vi "ADIS16448 IMU Example.vi"() -> ()   [LabVIEW 2019]
uses:
  <vilib>/Utility/RT CPU Load.ctl
  ADIS16448Lib/Typedef/ADIS16448 Hardware Configuration.ctl
  <vilib>/Rock Robotics/WPI/SPI/WPI_SPIMode.ctl
  <vilib>/Rock Robotics/SystemInterfaces/DIO/FPGA_DIOChannel.ctl
  <vilib>/Rock Robotics/SystemInterfaces/spilib/spi_bus.ctl
  <vilib>/NI_Real-Time Target Support.lvlib
panel:
  out "Accelerometers":T1(graph)
  out "IMU Detected?":bool
  in  "Calibration Time (sec)":u32=4
  in  "Hardware Config":T2={"SPI Clock Rate (Hz)"=1000000.0, "IMU SPI Mode (3)"=enum."Mode 3 (Clk Idle High,Sample on Trailing)", "IMU Reset Pin"=enum."DIO MXP 8", "IMU SPI Bus"=enum."SPI MXP", "IMU Data Ready Pin"=enum."DIO MXP 0", "Stall Config"={"Pow2BytesPerRead"=255, "StallTicks"=1000, "CsToSclkTicks"=5}, "IMU Status LED Pin"=enum."DIO MXP 9"}
  in  "Recalibrate?":bool
  in  "Reset?":bool
  out "Integrated Gyro Angle":T1(graph)
  out "Calibrated?":bool
  in  "Set Cal Time":bool
  out "CPU loads":T6[](array[typedef]) {"ISR (%)" format="%#.2f"; "Idle (%)" format="%#.2f"; "Background (%)" format="%#.2f"; "Normal (%)" format="%#.2f"; "Above Normal (%)" format="%#.2f"; "High (%)" format="%#.2g"; "Timed Structures (%)" format="%#.2g"; "Time Critical (%)" format="%#.2g"; "Total (%)" format="%#.2g"}
  in  "stop":bool
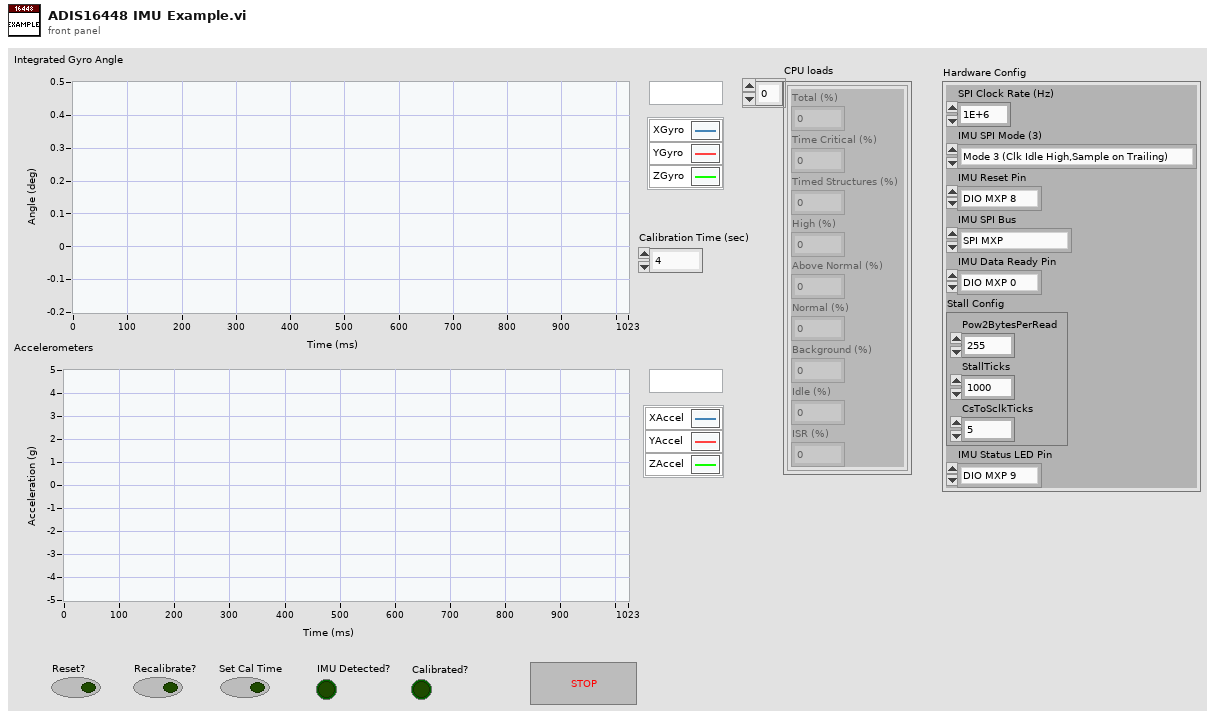
[diagram p1: front panel]
types:
  T1 = cluster{"XAngle":dbl, "YAngle":dbl, "ZAngle":dbl}
  T2 = typedef "ADIS16448 Hardware Configuration.ctl" = cluster{"SPI Clock Rate (Hz)":dbl, "IMU SPI Mode (3)":T3, "IMU Reset Pin":T4, "IMU SPI Bus":T5, "IMU Data Ready Pin":T4, "Stall Config":cluster{"Pow2BytesPerRead":u8, "StallTicks":u16, "CsToSclkTicks":u8}, "IMU Status LED Pin":T4}
  T3 = typedef "WPI_SPIMode.ctl" = enum16{"Mode 0 (Clk Idle Low,Sample on Leading)", "Mode 1 (Clk Idle Low,Sample on Trailing)", "Mode 2 (Clk Idle High,Sample on Leading)", "Mode 3 (Clk Idle High,Sample on Trailing)"}
  T4 = typedef "FPGA_DIOChannel.ctl" = enum8{"DIO 0", "DIO 1", "DIO 2", "DIO 3", "DIO 4", "DIO 5", "DIO 6", "DIO 7", "DIO 8", "DIO 9", "DIO MXP 0", "DIO MXP 1", "DIO MXP 2", "DIO MXP 3", "DIO MXP 4", "DIO MXP 5", "DIO MXP 6", "DIO MXP 7", "DIO MXP 8", "DIO MXP 9", "DIO MXP 10", "DIO MXP 11", "DIO MXP 12", "DIO MXP 13", "DIO MXP 14", "DIO MXP 15", "SPI Port CS1", "SPI Port CS2", "SPI Port CS3", "SPI Port MISO", "SPI Port MOSI", "Invalid"}
  T5 = typedef "spi_bus.ctl" = enum16{"SPI On-Board, CS0", "SPI On-Board, CS1", "SPI On-Board, CS2", "SPI On-Board, CS3", "SPI MXP", "Invalid"}
  T6 = typedef "NI_Real-Time Target Support.lvlib/RT CPU Load.ctl" = cluster{"Total (%)":dbl, "Time Critical (%)":dbl, "Timed Structures (%)":dbl, "High (%)":dbl, "Above Normal (%)":dbl, "Normal (%)":dbl, "Background (%)":dbl, "Idle (%)":dbl, "ISR (%)":dbl}
  T7 = typedef "ADIS16448 Device Reference.ctl" = cluster{"DevStatus":errorcluster, "Hardware Config":T2, "Calibration Complete":refnum<notifier>, "Status FIFO":refnum<k33>, "Last Value Reference":refnum<data-value>, "Sychronous Process VI":T8, "Cmd FIFO":refnum<k33>, "Source":T9, "Data FIFO":refnum<k33>, "IMU Status LED Pin":T4, "Calibration Time":u32}
  T8 = typedef "ADIS16448 Process.ctl" = refnum<vi>
  T9 = typedef "FPGA_CounterEncoderSourceConvertionLVSourceType.ctl" = cluster{"DevStatus":errorcluster, "AnalogTriggerMode?":bool, "DigitalMode":cluster{"DIO Channel":T10}, "AnalogTriggerMode":cluster{"AnalogTriggerIndex":T11, "OutputType":T12}}
  T10 = typedef "FPGA_DIODigitalSourceChannel.ctl" = enum8{"DIO 0", "DIO 1", "DIO 2", "DIO 3", "DIO 4", "DIO 5", "DIO 6", "DIO 7", "DIO 8", "DIO 9", "DIO MXP 0", "DIO MXP 1", "DIO MXP 2", "DIO MXP 3", "DIO MXP 4", "DIO MXP 5", "DIO MXP 6", "DIO MXP 7", "DIO MXP 8", "DIO MXP 9", "DIO MXP 10", "DIO MXP 11", "DIO MXP 12", "DIO MXP 13", "DIO MXP 14", "DIO MXP 15", "SPI Port CS1", "SPI Port CS2", "SPI Port CS3", "SPI Port MISO", "SPI Port MOSI", "Disabled"}
  T11 = typedef "FPGA_AnalogTriggerIndex.ctl" = enum8{"Trig 0", "Trig 1", "Trig 2", "Trig 3", "Trig 4", "Trig 5", "Trig 6", "Trig 7", "Invalid"}
  T12 = typedef "FPGA_AnalogTriggerOutType.ctl" = enum16{"InWindow", "TriggerState", "Rising", "Falling"}
  T13 = typedef "ADIS16448 Status.ctl" = cluster{"Calibrated?":bool, "IMU Detected?":bool}
  T14 = typedef "ADIS16448 Data.ctl" = cluster{"XAngle":dbl, "YAngle":dbl, "ZAngle":dbl, "XAcceleration":dbl, "YAcceleration":dbl, "ZAcceleration":dbl}
  T15 = cluster{"XAcceleration":dbl, "YAcceleration":dbl, "ZAcceleration":dbl}
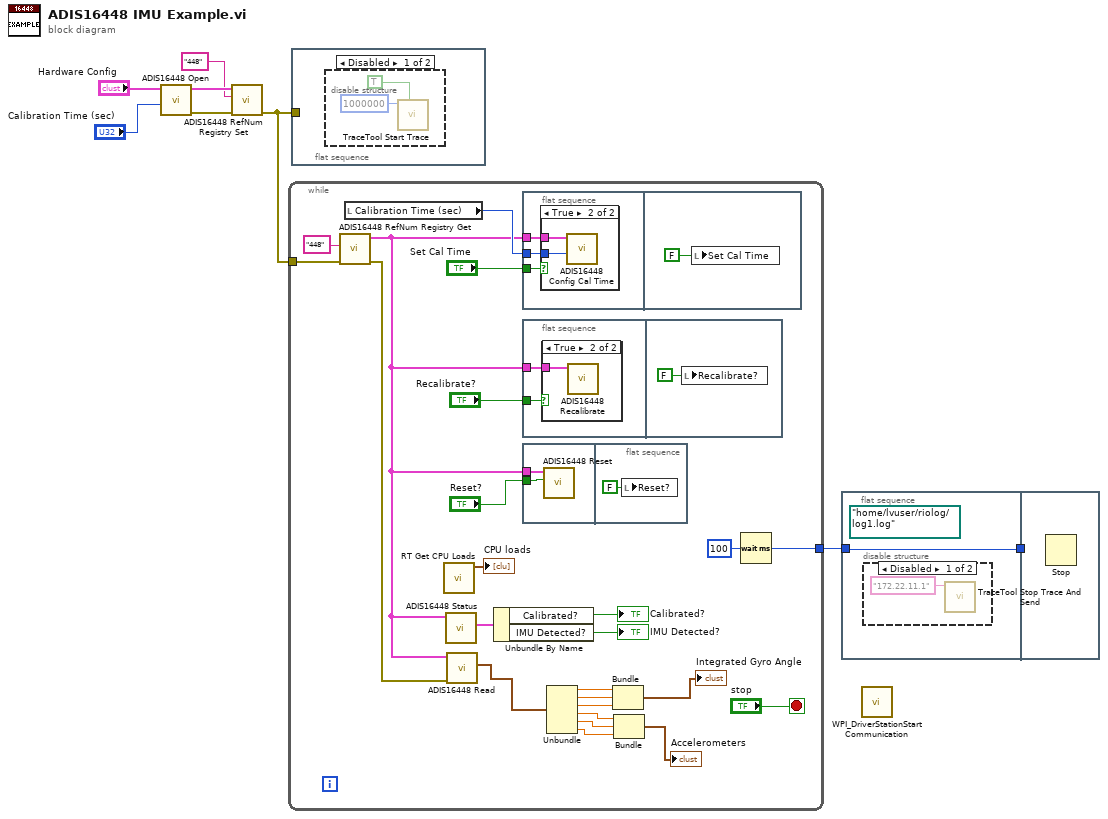
[diagram p0: block diagram]
diagram:
  n1 = call "ADIS16448 Open.vi"("Initial Calibration Time (sec)"="Calibration Time (sec)", "Hardware Config"="Hardware Config") -> ("error out"=w4:errorcluster, "ADIS16448DevRef"=w3:T7)  [unwired: 8 in]
  n2 = call "ADIS16448 RefNum Registry Set.vi"("error in (no error)"=w4, "refnum name"="448", "ADIS16448DevRef"=w3) -> ("error out"=w1:errorcluster)  [unwired: 7 in, 1 out]
  n3 = while {
    tunnel: [w29] -> w8
    tunnel: w1 -> [w19]
    stop <- "stop" stop-if-true
    n4 = call "ADIS16448 RefNum Registry Get.vi"("error in (no error)"=w19, "refnum name"="448") -> ("error out"=w18:errorcluster, "ADIS16448DevRef Out"=w21:T7)  [unwired: 8 in]
    n5 = local read "Calibration Time (sec)"() -> (w23:u32)
    n6 = call <vilib>:"RT Get CPU Loads.vi"() -> ("CPU loads"=→"CPU loads":T6[])  [unwired: 10 in, 1 out]
    n7 = call "ADIS16448 Status.vi"("ADIS16448DevRef"=w21) -> ("ADIS16448 Status"=w27:T13)  [unwired: 8 in, 2 out]
    n8 = call "ADIS16448 Read.vi"("error in (no error)"=w18, "ADIS16448DevRef"=w21) -> ("ADIS16448 Value"=w17:T14)  [unwired: 6 in, 3 out]
    n9 = Unbundle By Name(w27) -> ("Calibrated?"=→"Calibrated?":bool, "IMU Detected?"=→"IMU Detected?":bool)
    n10 = flat-sequence {
      tunnel: "Set Cal Time" -> [w35]
      tunnel: w23 -> [w34]
      tunnel: w21 -> [w33]
      frame #0 {
        n11 = case shown="True" w35 {
          tunnel: w34 -> [_ w37]
          tunnel: w33 -> [_ w36]
          frame False {
          }
          frame True {
            n12 = call "ADIS16448 Config Cal Time.vi"("Data"=w37, "ADIS16448DevRef in"=w36) -> ()  [unwired: 8 in, 2 out]
          }
        }
      }
      frame #1 {
        n13 = local write "Set Cal Time"(FALSE ("Ready?")) -> ()
      }
    }
    n14 = flat-sequence {
      tunnel: "Recalibrate?" -> [w40]
      tunnel: w21 -> [w39]
      frame #0 {
        n15 = case shown="True" w40 {
          tunnel: w39 -> [_ w41]
          frame False {
          }
          frame True {
            n16 = call "ADIS16448 Recalibrate.vi"("ADIS16448DevRef in"=w41) -> ()  [unwired: 9 in, 2 out]
          }
        }
      }
      frame #1 {
        n17 = local write "Recalibrate?"(FALSE ("Recalibrate?")) -> ()
      }
    }
    n18 = flat-sequence {
      tunnel: "Reset?" -> [w44]
      tunnel: w21 -> [w43]
      frame #0 {
        n19 = call "ADIS16448 Reset.vi"("Reset?"=w44, "ADIS16448DevRef"=w43) -> ()  [unwired: 8 in, 2 out]
      }
      frame #1 {
        n20 = local write "Reset?"(FALSE ("Reset?")) -> ()
      }
    }
    n21 = Unbundle(w17) -> ("XAngle"=w16:dbl, "YAngle"=w15:dbl, "ZAngle"=w14:dbl, "XAcceleration"=w13:dbl, "YAcceleration"=w12:dbl, "ZAcceleration"=w11:dbl)
    n22 = Bundle("XAngle"=w16, "YAngle"=w15, "ZAngle"=w14) -> (→"Integrated Gyro Angle":T1)  [unwired: 1 in]
    n23 = Bundle("XAcceleration"=w13, "YAcceleration"=w12, "ZAcceleration"=w11) -> (→"Accelerometers":T15)  [unwired: 1 in]
    n24 = Wait (ms)(milliseconds to wait=u32 100) -> (millisecond timer value=w29:u32)
  }
  n25 = flat-sequence {
    tunnel: w1 -> [_]
    frame #0 {
      n26 = disable-structure shown="Disabled" {
        frame Disabled {
          n27 = call <vilib>:"TraceTool Start Trace.vi"("Detailed Tracing? (F)"=TRUE, "Buffer Size (250000 bytes)"=1000000) -> ()  [unwired: 8 in, 2 out]
        }
        frame Enabled {
        }
      }
    }
  }
  n28 = flat-sequence {
    tunnel: w8 -> [w48]
    tunnel: [w48] -> w7
    tunnel: w7 -> [_]
    frame #0 {
      (unwired) path "/home/lvuser/riolog/log1.log" ("Path to Trace Log")
      n29 = disable-structure shown="Disabled" {
        frame Disabled {
          n30 = call <vilib>:"TraceTool Stop Trace And Send.vi"("Trace Host Network Address"="172.22.11.1") -> ()  [unwired: 10 in, 1 out]
        }
        frame Enabled {
        }
      }
    }
    frame #1 {
      n31 = Stop() -> ()  [unwired: 1 in]
    }
  }
  n32 = call <vilib>:"WPI_DriverStationStart Communication.vi"() -> ()  [unwired: 12 in]
